vi "Eurotherm - Calculate Measured Reading.vi"(0 "Eurotherm Setup In":T1={"Communication"={"Com Port"=1, "Address"=1, "Baud Rate"=9600}, "Name"="", "Enable"=FALSE, "Max Set Point"=0.0, "Min Set Point"=0.0, "Units"="", "Graph Data"=0, "Sensor type"=enum."RhFe", "Calibration File Path"=path "", "Conversion Type"=enum."Linear"} {"Min Set Point" format="%.3f"; "Max Set Point" format="%.3f"; "Communication"."Baud Rate" items=["300"=300, "600"=600, "1200"=1200, "2400"=2400, "4800"=4800, "9600 (default)"=9600, "19200"=19200, "38400"=38400, "57600"=57600, "76800"=76800, "115200"=115200, "230400"=230400]; "Communication"."Com Port" min=1 max=255; "Communication"."Address" min=1 max=99}, 7 "Measured Value":dbl format="%.3f", 11 "error in (no error)":errorcluster) -> (4 "Eurotherm Setup Out":T1={"Communication"={"Com Port"=1, "Address"=1, "Baud Rate"=9600}, "Name"="", "Enable"=FALSE, "Max Set Point"=0.0, "Min Set Point"=0.0, "Units"="", "Graph Data"=0, "Sensor type"=enum."RhFe", "Calibration File Path"=path "", "Conversion Type"=enum."Linear"} {"Min Set Point" format="%.3f"; "Max Set Point" format="%.3f"; "Communication"."Baud Rate" items=["300"=300, "600"=600, "1200"=1200, "2400"=2400, "4800"=4800, "9600 (default)"=9600, "19200"=19200, "38400"=38400, "57600"=57600, "76800"=76800, "115200"=115200, "230400"=230400]; "Communication"."Com Port" min=1 max=255; "Communication"."Address" min=1 max=99}, 8 "Converted Value":dbl format="%.3f", 15 "error out":errorcluster)   [LabVIEW 2011]
uses:
  Eurotherm - Controls/Eurotherm - Setup.ctl
  Eurotherm - Controls/Eurotherm - Communication.ctl
  Common/Utilities/Controls - Com Ports/Com Port - Numeric.ctl
  Eurotherm - Controls/Eurotherm - Address.ctl
  Common/Utilities/Controls - Com Ports/Com Port - Baud Rate.ctl
  Common/Utilities - System/Sensors/Sensors - Controls/Sensors - Temperature Sensor Type.ctl
  Common/Utilities - System/Sensors/Sensors - Controls/Sensors - Conversion Type.ctl
  Common/Utilities - System/Sensors/Sensors - Controls/Sensors - Translation Type.ctl
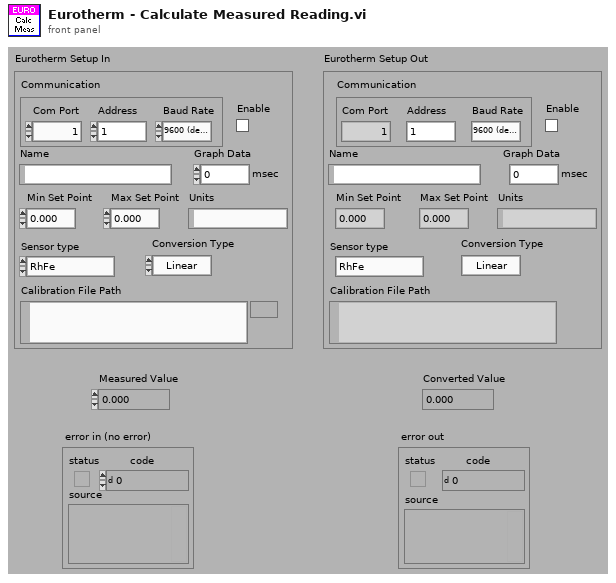
[diagram p1: front panel]
types:
  T1 = typedef "Eurotherm - Setup.ctl" = cluster{"Communication":T2, "Name":string, "Enable":bool, "Max Set Point":dbl, "Min Set Point":dbl, "Units":string, "Graph Data":u32, "Sensor type":T6, "Calibration File Path":path, "Conversion Type":T7}
  T2 = typedef "Eurotherm - Communication.ctl" = cluster{"Com Port":T3, "Address":T4, "Baud Rate":T5}
  T3 = typedef "Com Port - Numeric.ctl" = i32
  T4 = typedef "Eurotherm - Address.ctl" = u8
  T5 = typedef "Com Port - Baud Rate.ctl" = u32
  T6 = typedef "Sensors - Temperature Sensor Type.ctl" = enum16{"RhFe", "Pt", "K type thermocouple", "W5 type thermocouple", "No Conversion"}
  T7 = typedef "Sensors - Conversion Type.ctl" = enum16{"Linear", "Spline"}
  T8 = typedef "Sensors - Translation Type.ctl" = enum16{"K/C", "mV"}
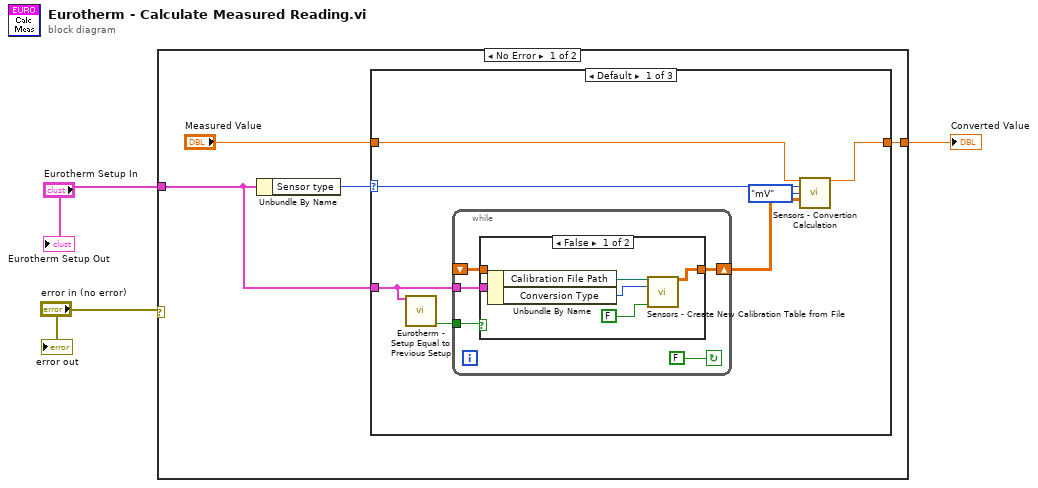
[diagram p0: block diagram]
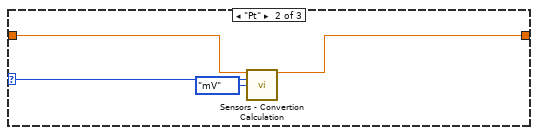
[diagram p3: hidden frame]
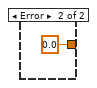
[diagram p5: hidden frame]
diagram:
  n1 = case shown="No Error" "error in (no error)" {
    tunnel: [w5 0.0] -> w3
    tunnel: "Eurotherm Setup In" -> [w4 _]
    frame No Error {
      n2 = Unbundle By Name(w4) -> ("Sensor type"=w7:T6)
      n3 = case shown="Default" w7 {
        selector: w7 -> [w12 w29 _]
        tunnel: "Measured Value" -> [w14 w27 w30]
        tunnel: [w13 w26 w30] -> w5
        tunnel: w4 -> [w10 _ _]
        frame Default {
          n4 = call "Eurotherm - Setup Equal to Previous Setup.vi"("Value In"=w10) -> ("Equal to previous value"=w9:bool)  [unwired: 13 in, 1 out]
          n5 = while {
            tunnel: w10 -> [w19]
            shift-right: [w18] -> w8
            shift-left: _ -> [w16]
            tunnel: w9 -> [w17]
            stop <- FALSE continue-if-true
            n6 = case shown="False" w17 {
              tunnel: w19 -> [w24 _]
              tunnel: [w20 w25] -> w18
              tunnel: w16 -> [_ w25]
              frame False {
                n7 = Unbundle By Name(w24) -> ("Calibration File Path"=w23:path, "Conversion Type"=w22:T7)
                n8 = call "Sensors - Create New Calibration Table from File.vi"("Calibration Data File"=w23, "Conversion Type"=w22, "Write table to file"=FALSE) -> ("Output Table"=w20:dbl[][])  [unwired: 12 in]
              }
              frame True {
              }
            }
          }
          n9 = call "Sensors - Convertion Calculation.vi"("Input Value"=w14, "Sensor type"=w12, "Translate To"=Sensors_-_Translation_Type."mV", "Input Table"=w8) -> ("Output Value"=w13:dbl)  [unwired: 10 in, 1 out]
        }
        frame "Pt" {
          n10 = call "Sensors - Convertion Calculation.vi"("Input Value"=w27, "Sensor type"=w29, "Translate To"=Sensors_-_Translation_Type."mV") -> ("Output Value"=w26:dbl)  [unwired: 11 in, 1 out]
        }
        frame "No Conversion" {
        }
      }
    }
    frame Error {
    }
  }
  "Converted Value" <- w3
  "error out" <- "error in (no error)"
  "Eurotherm Setup Out" <- "Eurotherm Setup In"
